vi "Read Drive Resolvers.vi"(1 "Input Array":dbl[](array[numeric])) -> (0 "Appended Array":dbl[](array[numeric]))   [LabVIEW 2014]
uses:
  Begin/Global RefNums.vi
  Begin/Global Constants.vi
panel:
  out "Drive Resolver BR":dbl
  out "Drive Resolver BL":dbl
  out "Drive Resolver FR":dbl
  out "Drive Resolver FL":dbl
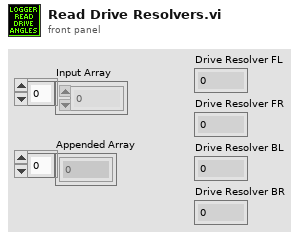
[diagram p1: front panel]
types:
  T1 = typedef "WPI_AnalogChannelDevRef.ctl" = cluster{"DevStatus":errorcluster, "Controller":T2, "Analog Channel":T3}
  T2 = typedef "FPGA_TypedefAnalogModule.ctl" = enum16{"Controller 1"}
  T3 = typedef "FPGA_AIChannel.ctl" = enum8{"AI 0", "AI 1", "AI 2", "AI 3", "AI MXP 0", "AI MXP 1", "AI MXP 2", "AI MXP 3", "Invalid"}
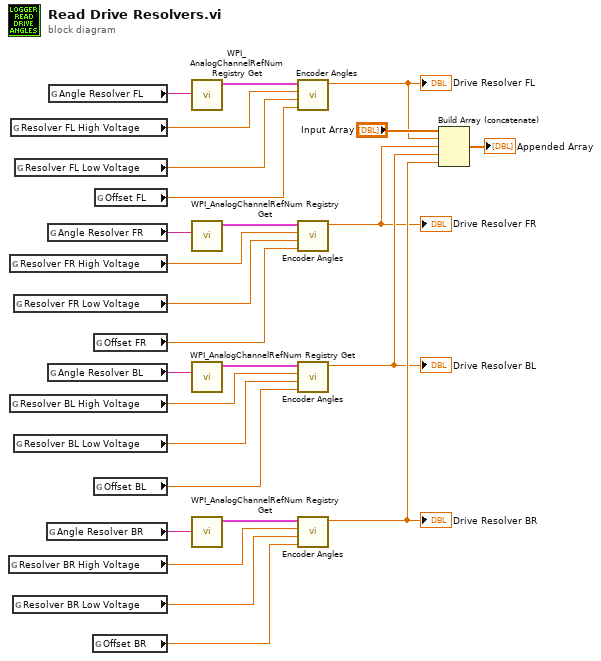
[diagram p0: block diagram]
diagram:
  n1 = global read "Global Constants.vi" "Resolver BR High Voltage"() -> (w19:dbl)
  n2 = global read "Global Constants.vi" "Resolver FR High Voltage"() -> (w15:dbl)
  n3 = global read "Global Constants.vi" "Resolver BL High Voltage"() -> (w21:dbl)
  n4 = global read "Global Constants.vi" "Resolver FL High Voltage"() -> (w17:dbl)
  n5 = global read "Global Constants.vi" "Resolver BR Low Voltage"() -> (w20:dbl)
  n6 = global read "Global Constants.vi" "Resolver FR Low Voltage"() -> (w16:dbl)
  n7 = global read "Global Constants.vi" "Resolver BL Low Voltage"() -> (w22:dbl)
  n8 = global read "Global Constants.vi" "Resolver FL Low Voltage"() -> (w18:dbl)
  n9 = global read "Global RefNums.vi" "Angle Resolver BR"() -> (w9:string)
  n10 = global read "Global RefNums.vi" "Angle Resolver FR"() -> (w7:string)
  n11 = global read "Global RefNums.vi" "Angle Resolver BL"() -> (w8:string)
  n12 = global read "Global RefNums.vi" "Angle Resolver FL"() -> (w10:string)
  n13 = global read "Global Constants.vi" "Offset BR"() -> (w25:dbl)
  n14 = global read "Global Constants.vi" "Offset FR"() -> (w23:dbl)
  n15 = global read "Global Constants.vi" "Offset BL"() -> (w26:dbl)
  n16 = global read "Global Constants.vi" "Offset FL"() -> (w24:dbl)
  n17 = call <vilib>:"WPI_AnalogChannelRefNum Registry Get.vi"("refnum name"=w10) -> ("AIDeviceRef"=w12:T1)  [unwired: 9 in, 1 out]
  n18 = call <vilib>:"WPI_AnalogChannelRefNum Registry Get.vi"("refnum name"=w7) -> ("AIDeviceRef"=w11:T1)  [unwired: 9 in, 1 out]
  n19 = call <vilib>:"WPI_AnalogChannelRefNum Registry Get.vi"("refnum name"=w8) -> ("AIDeviceRef"=w14:T1)  [unwired: 9 in, 1 out]
  n20 = call <vilib>:"WPI_AnalogChannelRefNum Registry Get.vi"("refnum name"=w9) -> ("AIDeviceRef"=w13:T1)  [unwired: 9 in, 1 out]
  n21 = call "Encoder Angles.vi"("calibration angle"=w24, "low voltage"=w18, "top voltage"=w17, "AIDeviceRef Encoder"=w12) -> ("encoder angle"=w4:dbl)  [unwired: 7 in]
  "Drive Resolver FL" <- w4
  n22 = call "Encoder Angles.vi"("calibration angle"=w23, "low voltage"=w16, "top voltage"=w15, "AIDeviceRef Encoder"=w11) -> ("encoder angle"=w1:dbl)  [unwired: 7 in]
  "Drive Resolver FR" <- w1
  n23 = call "Encoder Angles.vi"("calibration angle"=w26, "low voltage"=w22, "top voltage"=w21, "AIDeviceRef Encoder"=w14) -> ("encoder angle"=w2:dbl)  [unwired: 7 in]
  "Drive Resolver BL" <- w2
  n24 = call "Encoder Angles.vi"("calibration angle"=w25, "low voltage"=w20, "top voltage"=w19, "AIDeviceRef Encoder"=w13) -> ("encoder angle"=w3:dbl)  [unwired: 7 in]
  "Drive Resolver BR" <- w3
  n25 = Build Array (concatenate)("Input Array", w4, w1, w2, w3) -> (→"Appended Array":dbl[])
